vi "Messdaten TestRun Array.vi"(9 "Index":i32, 10 "Array (Eingang)":sgl[](array[numeric]), 11 "Array gesamt (Eingang)":sgl[][](array[numeric])) -> (3 "Array gesamt (Ausgang)":sgl[][](array[numeric]), 4 "Größe(n) ini":i32[](array[numeric]), 5 "Größe(n) Ausgang":i32[](array[numeric]), 6 "Größe Array":i32, 7 "Größe(n) Eingang":i32[](array[numeric]))   [LabVIEW 2020, in "EPA 1065.lvlib" / "HovaCAL Interference verificaton.lvlib"]
uses:
  HovaCAL Interference verificaton.lvlib
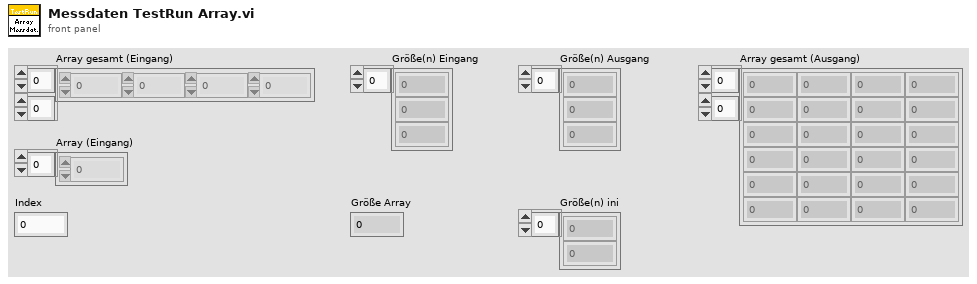
[diagram p1: front panel]
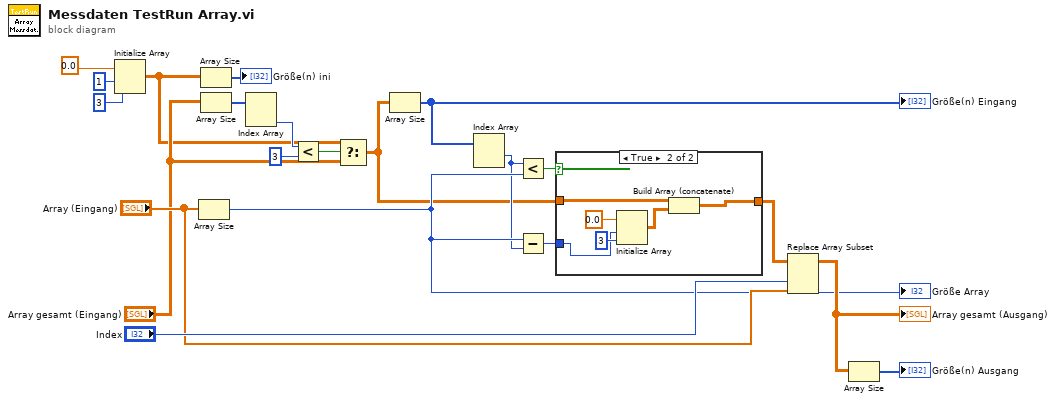
[diagram p0: block diagram]
diagram:
  n1 = Initialize Array(sgl 0.0 ("Numerisch"), 1 ("Dimensionsgröße"), 3 ("Dimensionsgröße")) -> (w8:sgl[][])
  n2 = Array Size(array="Array (Eingang)") -> (size(s)=w6:i32)
  "Größe Array" <- w6
  n3 = Array Size(array=w8) -> (size(s)=→"Größe(n) ini":i32[])
  n4 = Array Size(array="Array gesamt (Eingang)") -> (size(s)=w10:i32[])
  n5 = Index Array(array=w10) -> (element #2=w9:i32)  [unwired: 2 in, 1 out]
  n6 = Less?(x=w9, y=3) -> (x < y?=w16:bool)
  n7 = Select(t=w8, s=w16, f="Array gesamt (Eingang)") -> (s? t:f=w3:sgl[][])
  n8 = Array Size(array=w3) -> (size(s)=w11:i32[])
  "Größe(n) Eingang" <- w11
  n9 = Index Array(array=w11) -> (element #1=w5:i32)  [unwired: 2 in, 1 out]
  n10 = Less?(x=w5, y=w6) -> (x < y?=w4:bool)
  n11 = Subtract(x=w6, y=w5) -> (x-y=w2:i32)
  n12 = case shown="True" w4 {
    tunnel: w3 -> [w22 w25]
    tunnel: w2 -> [_ w26]
    tunnel: [w22 w23] -> w1
    frame False {
    }
    frame True {
      n13 = Initialize Array(sgl 0.0 ("Numerisch"), w26, 3 ("Dimensionsgröße")) -> (w24:sgl[][])
      n14 = Build Array (concatenate)(w25, w24) -> (w23:sgl[][])
    }
  }
  n15 = Replace Array Subset(array=w1, new element="Array (Eingang)", index (col)="Index") -> (w19:sgl[][])  [unwired: 1 in]
  "Array gesamt (Ausgang)" <- w19
  n16 = Array Size(array=w19) -> (size(s)=→"Größe(n) Ausgang":i32[])
